vi "Panel.vi"(11 "Numeric Analog Panel in":refnum<class "Numeric Analog Panel.lvclass">) -> ()   [LabVIEW 2020, in "VolatusGUI.lvlib" / "Numeric Analog Panel.lvclass"]
uses:
  Numeric Analog Panel.lvclass
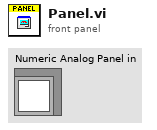
[diagram p1: front panel]
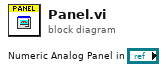
[diagram p0: block diagram]
diagram:
